vi "XML Script - GenericSubVI (Path).vi"(0 "name":string, 1 "prefix (name)":string, 2 "path":path, 3 "instantiation path":path, 5 "in":i32=-1, 8 "out":i32=-1) -> (6 "XML Script Command - SubVI":string, 9 "name (wire source)":string)   [LabVIEW 2020]
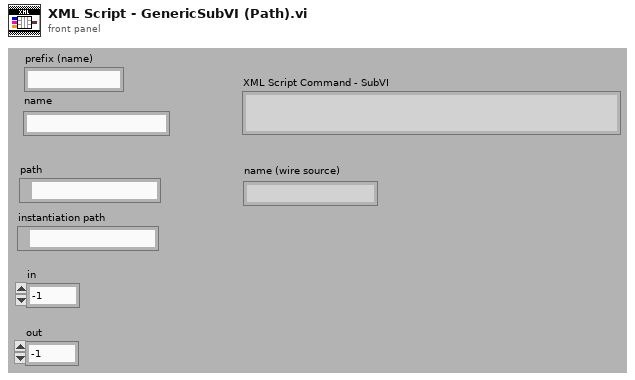
[diagram p1: front panel]
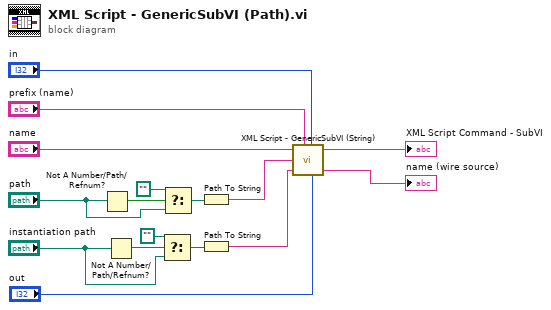
[diagram p0: block diagram]
diagram:
  n1 = Not A Number/Path/Refnum?(number/path/refnum="path") -> (NaN/Path/Refnum?=w3:bool)
  n2 = Not A Number/Path/Refnum?(number/path/refnum="instantiation path") -> (NaN/Path/Refnum?=w10:bool)
  n3 = Select(t=path "", s=w10, f="instantiation path") -> (s? t:f=w8:path)
  n4 = Select(t=path "", s=w3, f="path") -> (s? t:f=w5:path)
  n5 = Path To String(path=w5) -> (string=w1:string)
  n6 = Path To String(path=w8) -> (string=w6:string)
  n7 = call <vilib>:"XML Script - GenericSubVI (String).vi"("name"="name", "prefix (name)"="prefix (name)", "path"=w1, "instantiationPath"=w6, "in"="in", "out"="out") -> ("XML Script Command - SubVI"=→"XML Script Command - SubVI":string, "name (wire source)"=→"name (wire source)":string)  [unwired: 2 out]
